vi "LedState_Create.vi"(0 "reference in":refnum<class "LedState.lvclass">, 5 "error in (no error)":errorcluster) -> (14 "reference out":refnum<class "LedState.lvclass">, 19 "error out":errorcluster)   [LabVIEW 2014, in "LedState.lvclass"]
uses:
  LedState.lvclass
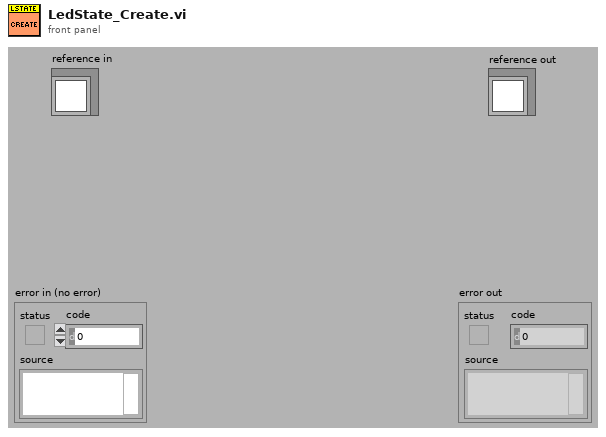
[diagram p1: front panel]
types:
  T1 = typedef "LedState.lvclass/ObjectAttributes.ctl" = cluster{"Led":bool}
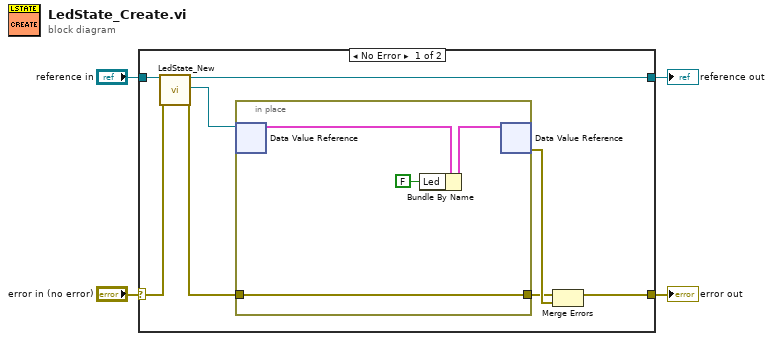
[diagram p0: block diagram]
diagram:
  n1 = case shown="No Error" "error in (no error)" {
    selector: "error in (no error)" -> [w11 w18]
    tunnel: [w8 w18] -> w3
    tunnel: "reference in" -> [w12 w17]
    tunnel: [w10 w17] -> w1
    frame No Error {
      n2 = call "LedState_New.vi"("reference in"=w12, "error in (no error)"=w11) -> ("reference out"=w10:refnum<class "LedState.lvclass">, "DVRRefOut"=w7:refnum<data-value>, "error out"=w6:errorcluster)  [unwired: 14 in, 1 out]
      n3 = in-place {
        in-place-border: w6 -> [w14]
        in-place-border: [w14] -> w5
        n4 = in-place-dvr #1(w7) -> (w15:T1)  [unwired: 1 out]
        n5 = Bundle By Name(cluster=w15, "Led"=FALSE) -> (w16:T1)
        n6 = in-place-dvr #1(w16) -> (w9:errorcluster)  [unwired: 1 out]
      }
      n7 = Merge Errors(w5, w9) -> (w8:errorcluster)
    }
    frame Error {
      # "VI-TechBaseTemplate_Simple_6x8x6"
    }
  }
  "error out" <- w3
  "reference out" <- w1
